vi "SignalReceiver.SetSetpoint.vi"(8 "error in (no error)":errorcluster, 10 "Setpoint":dbl, 11 "SignalReceiver":refnum<class "SignalReceiver.lvclass">) -> (0 "error out":errorcluster, 3 "SignalReceiver out":refnum<class "SignalReceiver.lvclass">)   [LabVIEW 2020, in "ECU_Diagnose.lvlib" / "SignalReceiver.lvclass"]
doc: "---------------------------------------------------------------\nJKI State Machine Objects™\nhttp://jki.net/state-machine-objects/\nCopyright (C) 2005-2015, JKI <info@jki.net>\nALL RIGHTS RESERVEDJKI State Machine Objects (SMO) 1.0.0.5\nJKI - JKI\nCopyright (c) 2016, JKI"
uses:
  SignalReceiver.lvclass
  Typedefs/SetpointChanged--EventData--Cluster.ctl
  Typedefs/Data.ctl
panel:
  # "For instructions on how to use the JKI State Machine Objects, examples and video tutorials, visit:\nhttp://jki.net/state-machine-objects/\n\nJKI State Machine Objects™\nhttp://jki.net/state-machine-objects/\nCopyright (C) 2005-2015, JKI <info@jki.net>\nALL RIGHTS RESERVED"
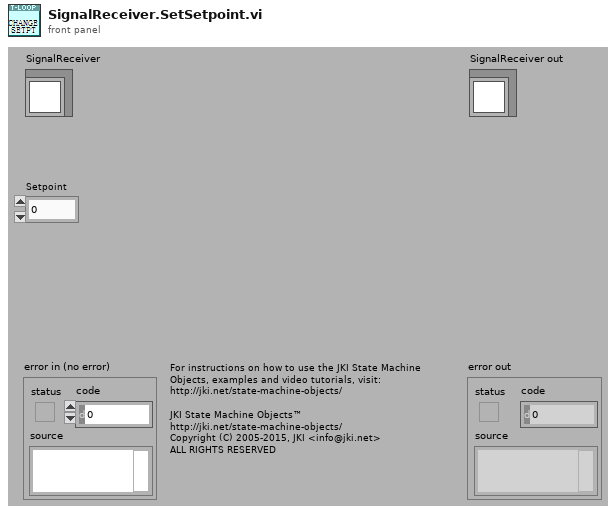
[diagram p1: front panel]
types:
  T1 = typedef "ECU_Diagnose.lvlib/SignalReceiver.lvclass/SetpointChanged--EventData--Cluster.ctl" = cluster{"Setpoint":T2}
  T2 = typedef "Data.ctl" = dbl
  T3 = typedef "ECU_Diagnose.lvlib/SignalReceiver.lvclass/PrivateData--Ref.ctl" = refnum<data-value>
  T4 = typedef "ECU_Diagnose.lvlib/SignalReceiver.lvclass/PrivateData--Cluster.ctl" = cluster{"Public Events":T5, "Private Events":T6, "SignalArrySelect":T7, "SignalDataReciArry":T8}
  T5 = typedef "ECU_Diagnose.lvlib/SignalReceiver.lvclass/PublicEvents--Cluster.ctl" = cluster{"Setpoint Changed":refnum<user-event>, "Value Changed":refnum<user-event>}
  T6 = typedef "ECU_Diagnose.lvlib/SignalReceiver.lvclass/PrivateEvents--Cluster.ctl" = cluster{"AsyncMethod":refnum<user-event>, "Start_Stop":refnum<user-event>}
  T7 = typedef "ECU_Diagnose.lvlib/SignalReceiver.lvclass/SignalArrySelecte.ctl" = cluster{"Port_No.":refnum<k21>, "XNET Signal":refnum<k21>[]}
  T8 = typedef "ECU_Diagnose.lvlib/SignalReceiver.lvclass/SignalDataArry.ctl" = cluster{"SignalDataReceiveArry":dbl[][], "Update":bool}
  T9 = typedef "SignalReceiver.lvclass/Data.ctl" = dbl
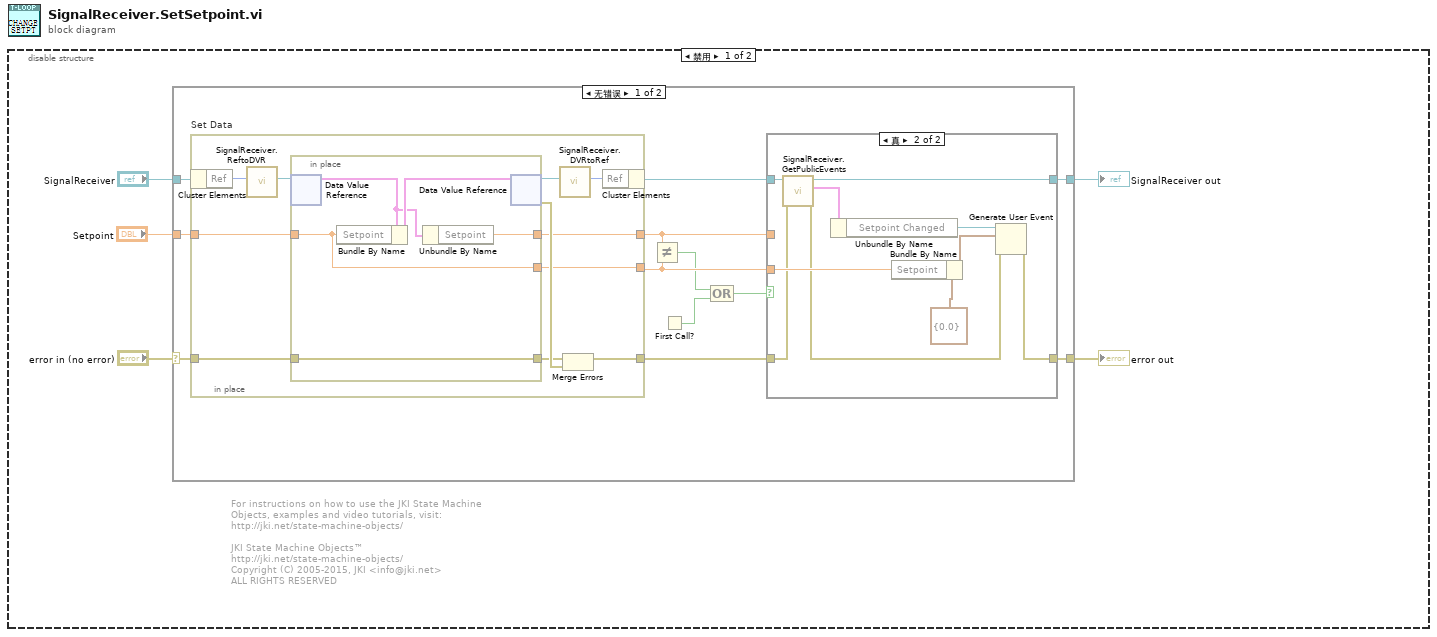
[diagram p0: block diagram]
diagram:
  n1 = disable-structure shown="禁用" {
    frame Disabled {
      # "For instructions on how to use the JKI State Machine Objects, examples and video tutorials, visit:\nhttp://jki.net/state-machine-objects/\n\nJKI State Machine Objects™\nhttp://jki.net/state-machine-objects/\nCopyright (C) 2005-2015, JKI <info@jki.net>\nALL RIGHTS RESERVED"
      n2 = case shown="无错误" "error in (no error)" {
        selector: "error in (no error)" -> [w15 w46]
        tunnel: "SignalReceiver" -> [w16 w47]
        tunnel: [w13 w46] -> w4
        tunnel: [w9 w47] -> w3
        tunnel: "Setpoint" -> [w17 _]
        frame No Error {
          n3 = in-place "Set Data" {
            in-place-border: w15 -> [w40]
            in-place-border: [w37] -> w14
            in-place-border: w17 -> [w36]
            in-place-border: [w35] -> w10
            in-place-border: [w34] -> w11
            n4 = in-place-cluster #1(w16) -> ("Ref"=w33:u32)
            n5 = call "SignalReceiver.ReftoDVR.vi"("Ref"=w33) -> ("Ref"=w32:T3)  [unwired: 10 in]
            n6 = in-place {
              in-place-border: w40 -> [w45]
              in-place-border: [w45] -> w38
              in-place-border: w36 -> [w43]
              in-place-border: [w43] -> w35
              in-place-border: [w42] -> w34
              n7 = in-place-dvr #2(w32) -> (w41:T4)  [unwired: 1 out]
              n8 = Bundle By Name(cluster=w41, "Setpoint"=w43) -> (w44:T4)
              n9 = Unbundle By Name(w41) -> ("Setpoint"=w42:T9)
              n10 = in-place-dvr #2(w44) -> (w31:T3, w39:errorcluster)
            }
            n11 = call "SignalReceiver.DVRtoRef.vi"("Ref"=w31) -> ("Ref"=w30:u32)  [unwired: 10 in]
            n12 = Merge Errors(w38, w39) -> (w37:errorcluster)
            n13 = in-place-cluster #1("Ref"=w30) -> (w12:refnum<class "SignalReceiver.lvclass">)
          }
          n14 = Not Equal?(x=w11, y=w10) -> (x != y?=w8:bool)
          n15 = First Call?() -> (First Call?: T/F=w7:bool)
          n16 = Compound Arithmetic op=OR(w8, w7) -> (w6:bool)
          n17 = case shown="真" w6 {
            tunnel: w14 -> [w18 w23]
            tunnel: w11 -> [_ _]
            tunnel: w10 -> [_ w26]
            tunnel: [w18 w25] -> w13
            tunnel: w12 -> [w19 w24]
            tunnel: [w19 w21] -> w9
            frame False {
            }
            frame True {
              n18 = call "SignalReceiver.GetPublicEvents.vi"("error in (no error)"=w23, "SignalReceiver"=w24) -> ("error out"=w22:errorcluster, "my Public Events"=w20:T5, "SignalReceiver out"=w21:refnum<class "SignalReceiver.lvclass">)  [unwired: 7 in]
              n19 = Unbundle By Name(w20) -> ("Setpoint Changed"=w29:refnum<user-event>)
              n20 = Bundle By Name(cluster=T1 {"Setpoint"=0.0} ("event data"), "Setpoint"=w26) -> (w27:T1)
              n21 = Generate User Event(user event=w29, event data cluster=w27, error in=w22) -> (error out=w25:errorcluster)  [unwired: 1 in, 1 out]
            }
          }
        }
        frame Error {
        }
      }
      "error out" <- w4
      "SignalReceiver out" <- w3
    }
    frame Enabled {
    }
  }
